vi "Truly Empty Almost Empty String Array.vi"(7 "String Array":string[](array[string])) -> (8 "String Array":string[](array[string]))   [LabVIEW 2021, in "Strings.lvlib"]
doc: "This VI deals with \"almost\" empty string arrays, where the array contains one or more empty strings and remove those strings.\n\nIn particular, it helps with the dreaded \"almost empty\" string array consisting of a single element which is empty. This is not considered an empty array in a test. This VI returns an empty array."
uses:
  Strings.lvlib
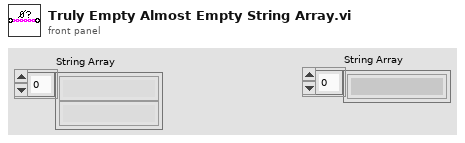
[diagram p1: front panel]
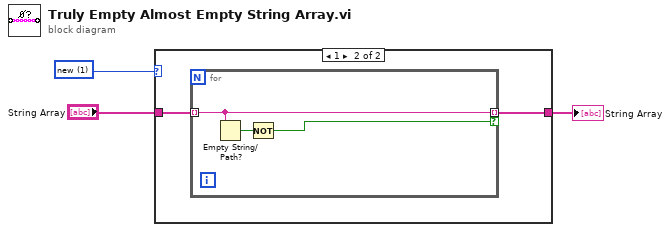
[diagram p0: block diagram]
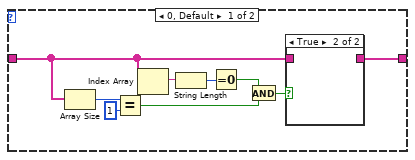
[diagram p2: hidden frame]
diagram:
  w1 = u16 1 items=["old", "new"]
  n1 = case shown="1" w1 {
    tunnel: [w12 w14] -> w3
    tunnel: "String Array" -> [w11 w15]
    frame 0, Default {
      n2 = Array Size(array=w11) -> (size(s)=w10:i32)
      n3 = Equal?(x=w10, y=1) -> (x = y?=w5:bool)
      n4 = Index Array(array=w11) -> (element=w8:string)  [unwired: 1 in]
      n5 = String Length(string=w8) -> (length=w7:i32)
      n6 = Equal To 0?(x=w7) -> (x = 0?=w6:bool)
      n7 = And(x=w6, y=w5) -> (x .and. y?=w4:bool)
      n8 = case shown="True" w4 {
        tunnel: w11 -> [w13 _]
        tunnel: [w13 _] -> w12
        frame False {
        }
        frame True {
        }
      }
    }
    frame 1 {
      n9 = for {
        tunnel: w15 -> [w18] mode=indexing
        tunnel: [w18] -> w14 mode=indexing if=w16
        n10 = Empty String/Path?(string/path=w18) -> (empty?=w17:bool)
        n11 = Not(x=w17) -> (.not. x?=w16:bool)
      }
    }
  }
  "String Array" <- w3
